vi "Gain Estimator.vi"(8 "error in (no error)":errorcluster) -> (0 "Error Out":errorcluster, 2 "Gain Out":dbl min=-50.0 max=50.0 step=1.0, 3 "Microphone Sensitvity (dBV/Pa) Out":dbl format="%#_13g")   [LabVIEW 2018, in "MainVIs.lvlib"]
uses:
  MainVIs.lvlib
  CollectionSupport.lvlib
panel:
  out "SPL":dbl
  in  "Gain":dbl min=-50.0 max=50.0 step=1.0
  in  "Microphone\n Sensitvity (dBV/Pa)":dbl format="%#_13g"
  in  "stop (F)":bool
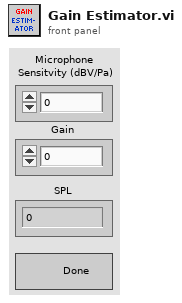
[diagram p1: front panel]
types:
  T1 = enum16{"open", "replace", "create", "open or create", "replace or create", "replace or create with confirmation"}
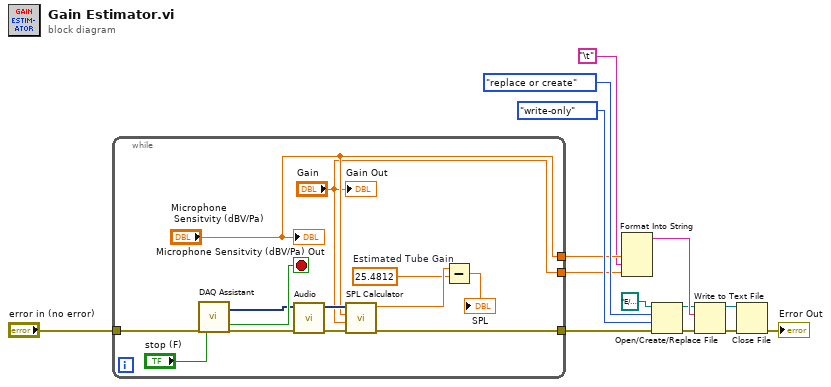
[diagram p0: block diagram]
diagram:
  n1 = while {
    tunnel: "error in (no error)" -> [w23]
    tunnel: [w20] -> w13
    tunnel: ["Microphone\n Sensitvity (dBV/Pa)"] -> w9
    tunnel: ["Gain"] -> w7
    stop <- w26 stop-if-true
    w15 = 25.4812  # Estimated Tube Gain
    n2 = call "DAQ Assistant"("error in"=w23, "stop (F)"="stop (F)") -> ("data"=w25:dynamicdata, "stopped"=w26:bool, "error out"=w22:errorcluster)  [unwired: 14 in, 1 out]
    n3 = call "Audio"("error in (no error)"=w22, "Signal"=w25) -> ("error out"=w21:errorcluster, "Filtered Signal"=w24:dynamicdata)  [unwired: 8 in]
    n4 = call "SPL Calculator.vi"("Error In"=w21, "Gain"="Gain", "Microphone Sensitvity (dBV/Pa)"="Microphone\n Sensitvity (dBV/Pa)", "Filtered Signal"=w24) -> ("Error Out"=w20:errorcluster, "SPL"=w16:dbl)  [unwired: 6 in]
    n5 = Subtract(x=w16, y=w15) -> (x-y=→"SPL":dbl)
    "Microphone Sensitvity (dBV/Pa) Out" <- "Microphone\n Sensitvity (dBV/Pa)"
    "Gain Out" <- "Gain"
  }
  n6 = Format Into String(w9, "\t", w7) -> (resulting string=w10:string)  [unwired: 3 in, 1 out]
  n7 = Open/Create/Replace File(file path (use dialog)=path "E:/Program Files/Master Aero Program/Calibration .txt files/SPL Gain.txt", error in=w13, operation (0:open)=T1."replace or create", access (0:read/write)=enum16{"read/write", "read-only", "write-only"}."write-only") -> (refnum out=w5:refnum<file>, error out=w2:errorcluster)  [unwired: 2 in, 1 out]
  n8 = Write to Text File(file (use dialog)=w5, text=w10, error in=w2) -> (refnum out=w1:refnum<file>, error out=w3:errorcluster)  [unwired: 1 in, 1 out]
  n9 = Close File(refnum=w1, error in=w3) -> (error out=→"Error Out":errorcluster)  [unwired: 1 out]
